vi "array_ends.vi"(11 "freqs_Hz":dbl[](array[numeric])) -> (3 "Array":dbl[](array[numeric]))   [LabVIEW 2017]
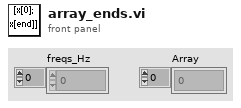
[diagram p1: front panel]
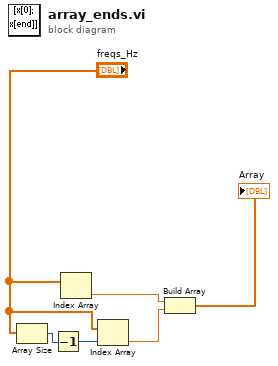
[diagram p0: block diagram]
diagram:
  n1 = Array Size(array="freqs_Hz") -> (size(s)=w4:i32)
  n2 = Decrement(x=w4) -> (x-1=w3:i32)
  n3 = Index Array(array="freqs_Hz") -> (element=w2:dbl)  [unwired: 1 in]
  n4 = Index Array(array="freqs_Hz", index=w3) -> (element=w1:dbl)
  n5 = Build Array(w2, w1) -> (→"Array":dbl[])
